vi "JustReadBuffer.vi"() -> ()   [LabVIEW 2014]
panel:
  in  "error in (no error)":errorcluster
  out "error out":errorcluster
  out "String 4":string
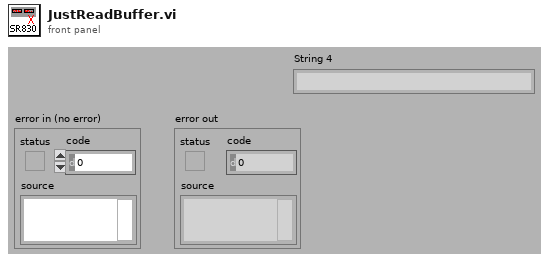
[diagram p1: front panel]
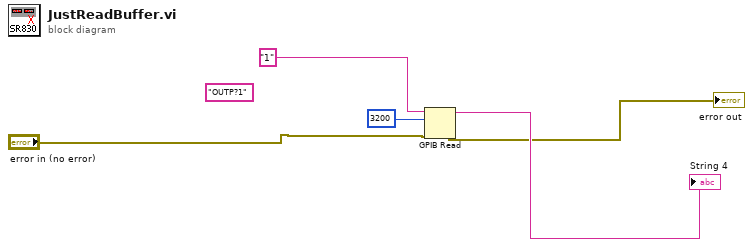
[diagram p0: block diagram]
diagram:
  (unwired) "OUTP?1"
  n1 = GPIB Read(0:"1", 1:3200, 3:"error in (no error)") -> (5:→"String 4":string, 7:→"error out":errorcluster)  [unwired: 2 in, 1 out]
